vi "Error - Top VI.vi"(8 "error in":errorcluster) -> (0 "error out":errorcluster)   [LabVIEW 2024, in "Error Handler.lvlib"]
uses:
  Error Handler.lvlib
  Error Queue - Dequeue.vi
  Support/User Events/User Events - Fire Error Event.vi
  Error Queue - Enqueue.vi
  Error Queue - Destroy.vi
  Support/User Events/User Events.lvlib
  Support/General Type Defs/Queue Message.ctl
  Support/General Type Defs/General Type Definitions.lvlib
  Support/General Type Defs/Error Handler Data.ctl
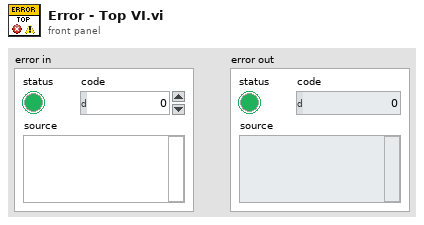
[diagram p1: front panel]
types:
  T1 = typedef "General Type Definitions.lvlib/Error Handler Data.ctl" = cluster{"Module":string, "Error Data":errorcluster, "Last Queue Message":T2}
  T2 = typedef "General Type Definitions.lvlib/Queue Message.ctl" = cluster{"Message":string, "Value":variant}
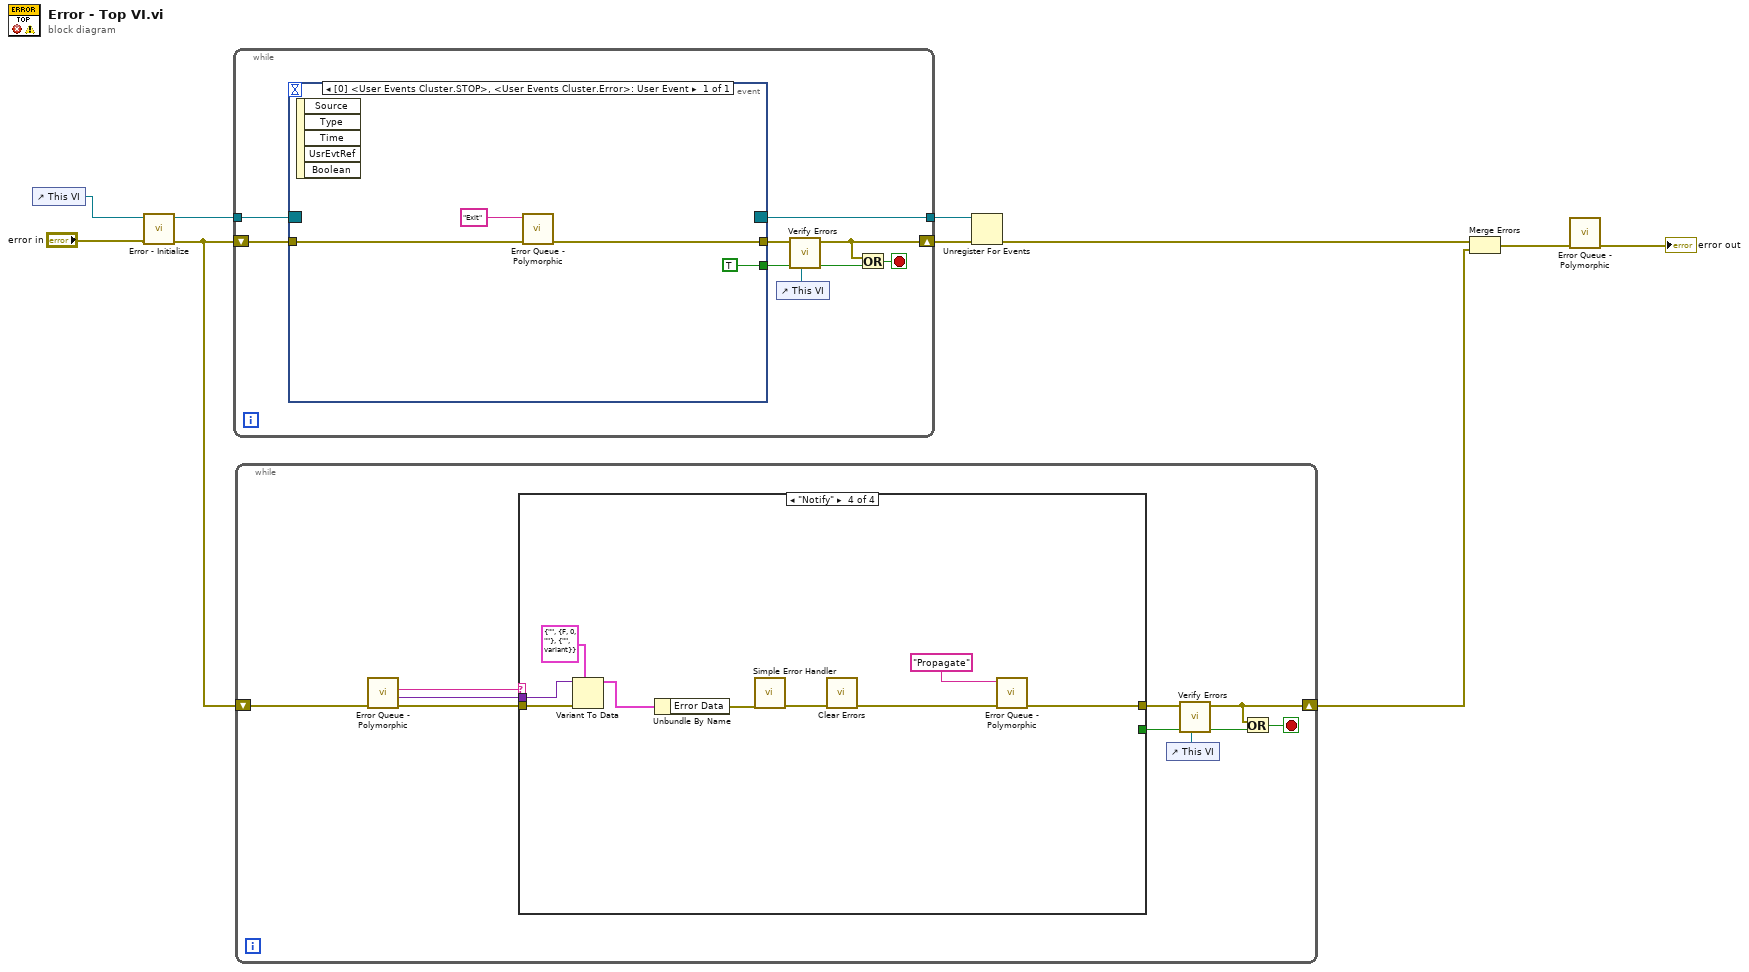
[diagram p0: block diagram]
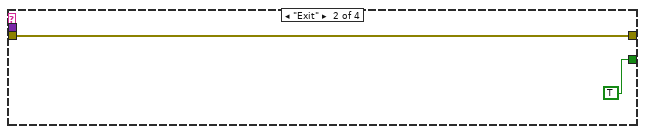
[diagram p3: hidden frame]
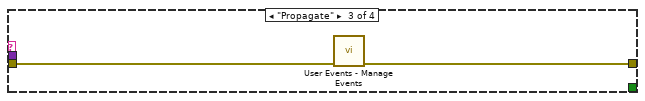
[diagram p4: hidden frame]
diagram:
  n1 = control-ref of="This VI"() -> (w10:refnum<vi>)
  n2 = call "Error - Initialize.vi"("error in (no error)"="error in", "VI In"=w10) -> ("error out"=w5:errorcluster, "Event Registration Out"=w8:refnum<event-registration>)  [unwired: 8 in]
  n3 = while {
    tunnel: w8 -> [w19]
    shift-right: [w14] -> w7
    shift-left: w5 -> [w18]
    tunnel: [w17] -> w6
    stop <- w16 stop-if-true
    n4 = event shown="[0] <User Events Cluster.STOP>, <User Events Cluster.Error>: User Event" {
      selector: w19 -> [_]
      dyn-events: [_] -> w17
      timeout: _ -> [_]
      tunnel: w18 -> [w23]
      tunnel: [w22] -> w15
      tunnel: [TRUE] -> w12
      event User Event {
        n5 = event-data() -> ()  [unwired: 1 in, 5 out]
        n6 = call-poly "Error Queue - Polymorphic.vi"("error in"=w23, "Message"="Exit") -> ("error out"=w22:errorcluster)  [unwired: 9 in]
      }
    }
    n7 = control-ref of="This VI"() -> (w13:refnum<vi>)
    n8 = call "Verify Errors.vi"("This VI"=w13, "STOP In"=w12, "error in"=w15) -> ("STOP Out"=w11:bool, "error out"=w14:errorcluster)  [unwired: 7 in]
    n9 = Or(x=w14, y=w11) -> (x .or. y?=w16:bool)
  }
  n10 = while {
    shift-right: [w27] -> w3
    shift-left: w5 -> [w33]
    stop <- w29 stop-if-true
    n11 = call-poly "Error Queue - Polymorphic.vi"("error in"=w33) -> ("error out"=w30:errorcluster, "Message Data"=w31:variant, "Message"=w32:string)  [unwired: 8 in]
    n12 = case shown="\"Notify\"" w32 {
      tunnel: w31 -> [_ _ _ w46]
      tunnel: w30 -> [w34 w35 w38 w47]
      tunnel: [w34 w35 w37 w43] -> w28
      tunnel: [_ TRUE _ _] -> w26
      frame "IDLE", Default {
      }
      frame "Exit" {
      }
      frame "Propagate" {
        n13 = call-poly "User Events - Manage Events.vi"("error in"=w38) -> ("error out"=w37:errorcluster)  [unwired: 10 in]
      }
      frame "Notify" {
        n14 = Variant To Data(error in=w47, type=T1 {"Module"="", "Error Data"={"status"=FALSE, "code"=0, "source"=""}, "Last Queue Message"={"Message"="", "Value"=variant}} ("Error Handler Data"), Variant=w46) -> (data=w40:T1)  [unwired: 1 out]
        n15 = Unbundle By Name(w40) -> ("Error Data"=w39:errorcluster)
        n16 = call <vilib>:"Simple Error Handler.vi"("error in (no error)"=w39) -> ("error out"=w45:errorcluster)  [unwired: 4 in, 4 out]
        n17 = call <vilib>:"Clear Errors.vi"("error in (no error)"=w45) -> ("error out"=w44:errorcluster)  [unwired: 5 in, 1 out]
        n18 = call-poly "Error Queue - Polymorphic.vi"("error in"=w44, "Message"="Propagate") -> ("error out"=w43:errorcluster)  [unwired: 9 in]
      }
    }
    n19 = control-ref of="This VI"() -> (w24:refnum<vi>)
    n20 = call "Verify Errors.vi"("This VI"=w24, "STOP In"=w26, "error in"=w28) -> ("STOP Out"=w25:bool, "error out"=w27:errorcluster)  [unwired: 7 in]
    n21 = Or(x=w27, y=w25) -> (x .or. y?=w29:bool)
  }
  n22 = Unregister For Events(event registration refnum=w6, error in=w7) -> (error out=w4:errorcluster)
  n23 = Merge Errors(w4, w3) -> (w2:errorcluster)
  n24 = call-poly "Error Queue - Polymorphic.vi"("error in"=w2) -> ("error out"=→"error out":errorcluster)  [unwired: 10 in]
